vi "Invert Lidar X Axis.vi"(11 "Cartesian Lidar Data":cluster{"X":dbl, "Y":dbl}[](array[cluster])) -> (3 "Inverted Lidar Data":cluster{"X":dbl, "Y":dbl}[](array[cluster]))   [LabVIEW 2017]
panel:
  # "Because the lidar is upside down, the data coming out of the lidar is inverted on the X axis. Objects to the left of the robot appear with positive X values."
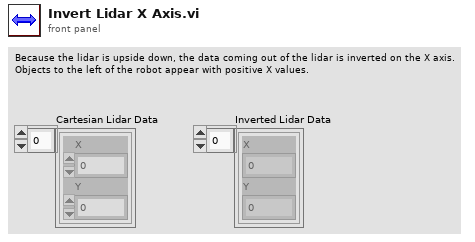
[diagram p1: front panel]
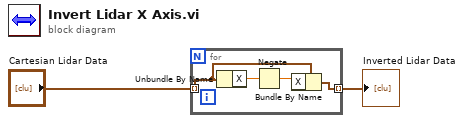
[diagram p0: block diagram]
diagram:
  n1 = for {
    tunnel: "Cartesian Lidar Data" -> [w4] mode=indexing
    tunnel: [w3] -> w2 mode=indexing
    n2 = Unbundle By Name(w4) -> ("X"=w6:dbl)
    n3 = Negate(x=w6) -> (-x=w5:dbl)
    n4 = Bundle By Name(cluster=w4, "X"=w5) -> (w3:cluster{"X":dbl, "Y":dbl})
  }
  "Inverted Lidar Data" <- w2
